vi "Measure Delta Mode.vi"(0 "Current Source Reference In":string="6221_GPIB12", 1 "Current Level (A)":dbl=1e-05, 2 "Current Range (A)":dbl=0.0001 format="%.2e", 3 "Current Source Compliance (V)":dbl=10.0 min=-1050.0 max=1050.0 step=1.0 format="%.4f", 5 "Voltmeter Reference In":refnum<visa-resource-name>="GPIB0::7::INSTR", 9 "Error in Current Source":errorcluster, 11 "Error In Voltmeter":errorcluster, 13 "Voltmeter Wait (ms)":u32=400) -> (4 "Current Source Reference Out":refnum<k15>, 6 "Voltmeter Reference Out":refnum<visa-resource-name>="GPIB0::7::INSTR", 8 "Resistance":dbl=1.1800557999999999, 10 "Error Out Current Source":errorcluster, 15 "Error Out Voltmeter":errorcluster)   [LabVIEW 2020]
uses:
  <instrlib>/Keithley 2182/Keithley 2182.lvlib
panel:
  out "Pulse Down Voltage":dbl=-2.087828e-05
  out "Pulse Up Voltage":dbl=2.722836e-06
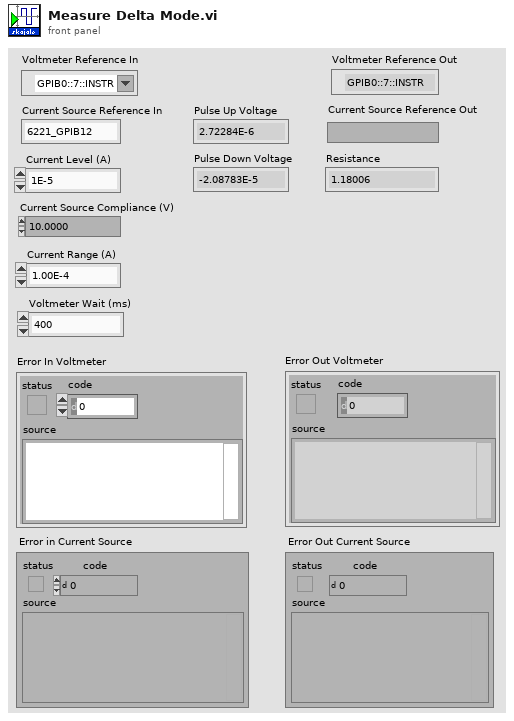
[diagram p1: front panel]
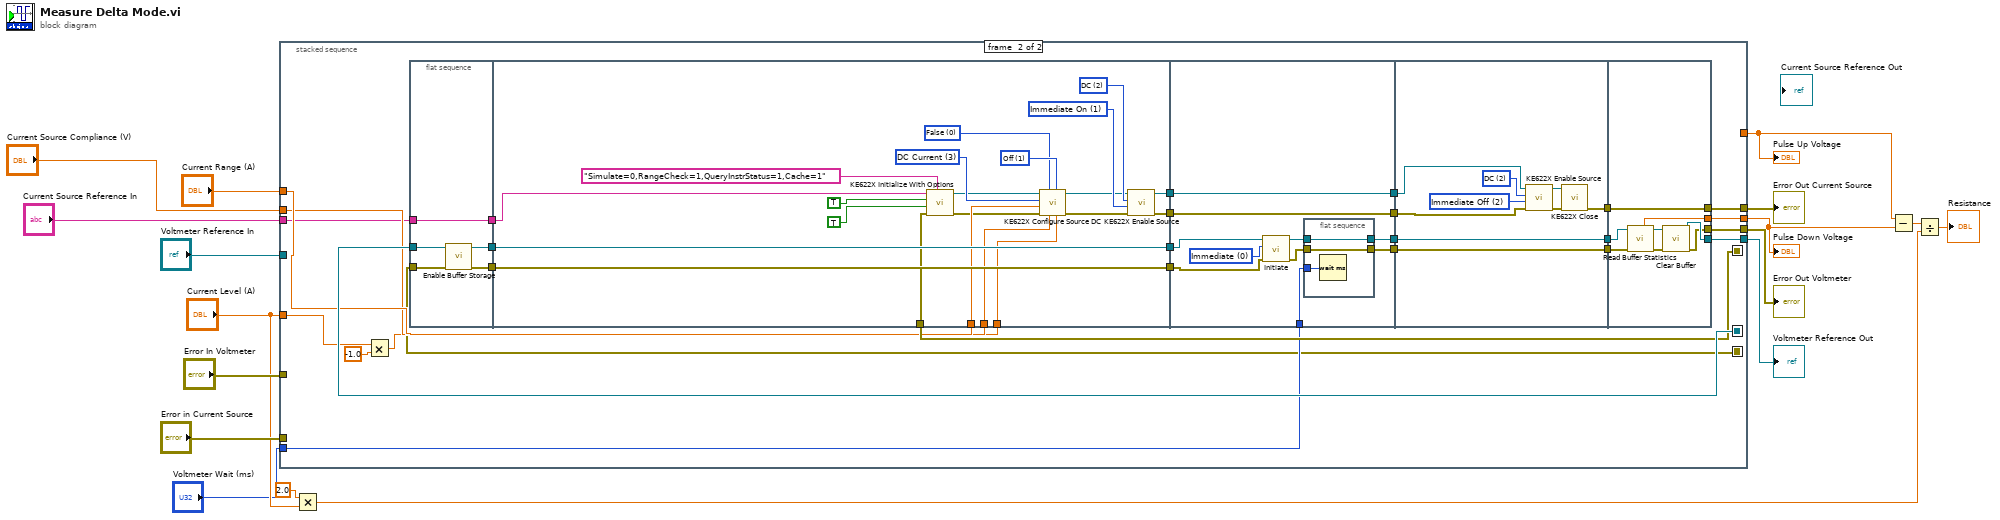
[diagram p0: block diagram]
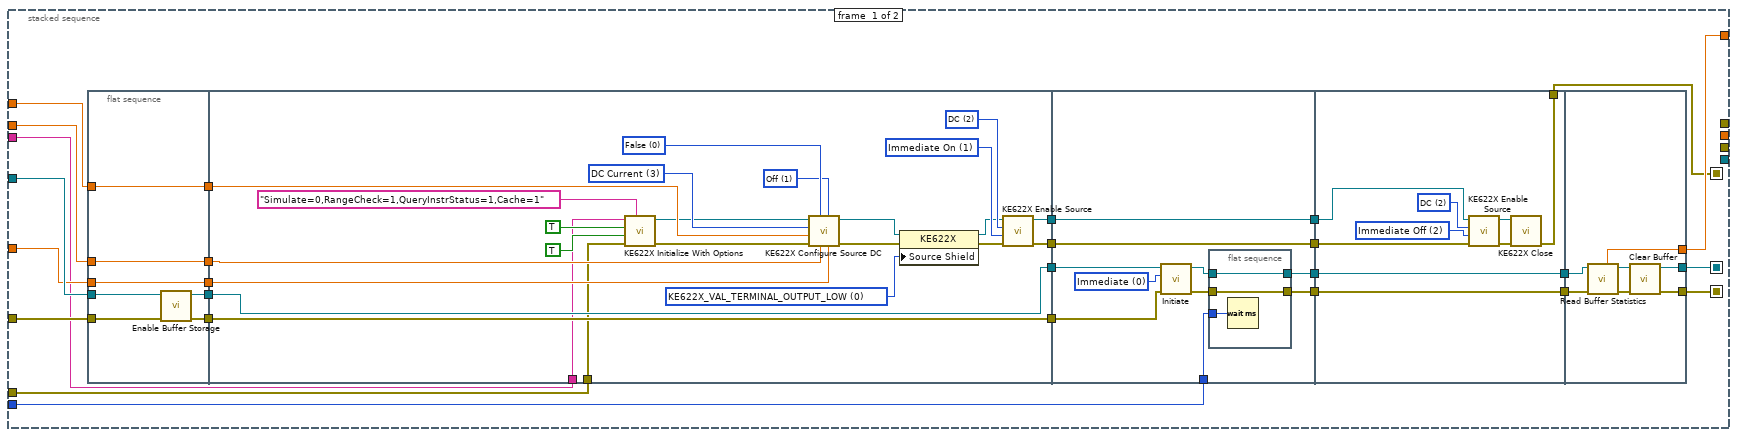
[diagram p2: hidden frame]
diagram:
  n1 = stacked-sequence {
    seq-local: [w31 _] -> [_ w120]
    seq-local: [w30 _] -> [_ w106]
    seq-local: [w29 _] -> [_ w119]
    tunnel: [w32 _] -> w15
    tunnel: [_ w118] -> w14
    tunnel: [_ w117] -> w4
    tunnel: [_ w116] -> w17
    tunnel: [_ w114] -> w16
    tunnel: "Voltmeter Reference In" -> [w28 _]
    tunnel: "Current Range (A)" -> [w26 w113]
    tunnel: "Error in Current Source" -> [w25 _]
    tunnel: "Current Source Compliance (V)" -> [w23 w112]
    tunnel: "Current Level (A)" -> [w22 w111]
    tunnel: "Error In Voltmeter" -> [w20 _]
    tunnel: "Voltmeter Wait (ms)" -> [w19 w108]
    tunnel: "Current Source Reference In" -> [w18 w105]
    frame #0 {
      n2 = flat-sequence {
        tunnel: [w51] -> w44
        tunnel: [w50] -> w43
        tunnel: w28 -> [w49]
        tunnel: w26 -> [w48]
        tunnel: [w48] -> w27
        tunnel: w23 -> [w47]
        tunnel: [w47] -> w24
        tunnel: w22 -> [w46]
        tunnel: [w46] -> w21
        tunnel: w20 -> [w45]
        tunnel: [w75] -> w42
        tunnel: w44 -> [w75]
        tunnel: [w74] -> w41
        tunnel: w43 -> [w74]
        tunnel: [w71] -> w40
        tunnel: [w70] -> w39
        tunnel: w27 -> [w66]
        tunnel: w25 -> [w56]
        tunnel: w24 -> [w65]
        tunnel: w21 -> [w64]
        tunnel: w18 -> [w52]
        tunnel: w42 -> [w83]
        tunnel: w41 -> [w82]
        tunnel: [w80] -> w38
        tunnel: [w79] -> w37
        tunnel: [w78] -> w36
        tunnel: w40 -> [w78]
        tunnel: [w77] -> w35
        tunnel: w39 -> [w77]
        tunnel: w19 -> [w76]
        tunnel: [w97] -> w34
        tunnel: w38 -> [w97]
        tunnel: [w96] -> w33
        tunnel: w37 -> [w96]
        tunnel: w36 -> [w95]
        tunnel: w35 -> [w94]
        tunnel: [w89] -> w29
        tunnel: w34 -> [w104]
        tunnel: w33 -> [w102]
        tunnel: [w100] -> w31
        tunnel: [w98] -> w32
        tunnel: [w99] -> w30
        frame #0 {
          n3 = call <instrlib>:"Enable Buffer Storage.vi"("error in (no error)"=w45, "VISA resource name"=w49) -> ("error out"=w50:errorcluster, "VISA resource name out"=w51:refnum<visa-resource-name>)  [unwired: 8 in]
        }
        frame #1 {
          w59 = 0 items=["KE622X_VAL_TERMINAL_OUTPUT_LOW", "KE622X_VAL_TERMINAL_GUARD"] ("System Settings:Source Shield")
          w67 = 3 items=["DC Current"=3] ("function")
          w68 = 1 items=["Off"=1, "HighZ"=3] ("standby mode")
          w69 = u16 0 items=["False"] ("enable pulsing")
          w72 = 1 items=["Immediate On"=1, "Immediate Off"=2, "Immediate Standby"=4, "Auto Sync Enabled"=65536, "Auto Sync Disabled"=131072, "Abort On Compliance Enabled"=16777216, "Abort On Compliance Disabled"=33554432] ("output action")
          w73 = 2 items=["Bias"=1, "Custom"=8, "DC"=2, "Sweep"=4, "Pulse Gen"=16, "Standard Waveform"=32, "Arbitrary Waveform"=64] ("generator")
          n4 = call <instrlib>:"KE622X Initialize With Options.vi"("option string"="Simulate=0,RangeCheck=1,QueryInstrStatus=1,Cache=1", "error in (no error)"=w56, "reset device"=TRUE, "id query"=TRUE, "resource name"=w52) -> ("error out"=w55:errorcluster, "instrument handle out"=w54:refnum<k15>)  [unwired: 5 in]
          n5 = call <instrlib>:"KE622X Configure Source DC.vi"("level"=w64, "standby mode"=w68, "compliance limit"=w65, "enable pulsing"=w69, "error in (no error)"=w55, "range"=w66, "function"=w67, "instrument handle"=w54) -> ("error out"=w62:errorcluster, "instrument handle out"=w63:refnum<k15>)  [unwired: 2 in]
          n6 = property class="KE622X"(reference=w63, error in=w62, "Source Shield"=w59) -> (reference out=w61:refnum<k15>, error out=w60:errorcluster)
          n7 = call <instrlib>:"KE622X Enable Source.vi"("error in (no error)"=w60, "output action"=w72, "generator"=w73, "instrument handle"=w61) -> ("error out"=w70:errorcluster, "instrument handle out"=w71:refnum<k15>)  [unwired: 6 in]
        }
        frame #2 {
          w81 = 0 items=["Immediate", "Continuous"] ("Initiate Type (0: Immediate)")
          n8 = call <instrlib>:"Initiate.vi"("error in (no error)"=w82, "Initiate Type (0: Immediate)"=w81, "VISA resource name"=w83) -> ("error out"=w85:errorcluster, "VISA resource name out"=w84:refnum<visa-resource-name>)  [unwired: 7 in]
          n9 = flat-sequence {
            tunnel: w76 -> [w88]
            tunnel: [w87] -> w79
            tunnel: w85 -> [w87]
            tunnel: [w86] -> w80
            tunnel: w84 -> [w86]
            frame #0 {
              n10 = Wait (ms)(milliseconds to wait=w88) -> ()  [unwired: 1 out]
            }
          }
        }
        frame #3 {
          w92 = 2 items=["Immediate On"=1, "Immediate Off"=2, "Immediate Standby"=4, "Auto Sync Enabled"=65536, "Auto Sync Disabled"=131072, "Abort On Compliance Enabled"=16777216, "Abort On Compliance Disabled"=33554432] ("output action")
          w93 = 2 items=["Bias"=1, "Custom"=8, "DC"=2, "Sweep"=4, "Pulse Gen"=16, "Standard Waveform"=32, "Arbitrary Waveform"=64] ("generator")
          n11 = call <instrlib>:"KE622X Enable Source.vi"("error in (no error)"=w94, "output action"=w92, "generator"=w93, "instrument handle"=w95) -> ("error out"=w90:errorcluster, "instrument handle out"=w91:refnum<k15>)  [unwired: 6 in]
          n12 = call <userlib>:"KE622X Close.vi"("error in (no error)"=w90, "instrument handle"=w91) -> ("error out"=w89:errorcluster)  [unwired: 9 in]
        }
        frame #4 {
          n13 = call <instrlib>:"Read Buffer Statistics.vi"("error in (no error)"=w102, "VISA resource name"=w104) -> ("error out"=w101:errorcluster, "VISA resource name out"=w103:refnum<visa-resource-name>, "Mean"=w98:dbl)  [unwired: 4 in, 3 out]
          n14 = call <instrlib>:"Clear Buffer.vi"("error in (no error)"=w101, "VISA resource name"=w103) -> ("error out"=w99:errorcluster, "VISA resource name out"=w100:refnum<visa-resource-name>)  [unwired: 8 in]
        }
      }
    }
    frame #1 {
      n15 = Multiply(x=w111, y=-1.0) -> (x*y=w109:dbl)
      n16 = flat-sequence {
        tunnel: [w137] -> w132
        tunnel: [w136] -> w131
        tunnel: w120 -> [w135]
        tunnel: w106 -> [w134]
        tunnel: [w133] -> w107
        tunnel: w105 -> [w133]
        tunnel: [w158] -> w130
        tunnel: w132 -> [w158]
        tunnel: [w157] -> w129
        tunnel: w131 -> [w157]
        tunnel: [w154] -> w128
        tunnel: [w153] -> w127
        tunnel: w119 -> [w142]
        tunnel: w113 -> [w147]
        tunnel: w112 -> [w146]
        tunnel: w109 -> [w145]
        tunnel: w107 -> [w143]
        tunnel: w130 -> [w166]
        tunnel: w129 -> [w165]
        tunnel: [w163] -> w126
        tunnel: [w162] -> w125
        tunnel: [w161] -> w124
        tunnel: w128 -> [w161]
        tunnel: [w160] -> w123
        tunnel: w127 -> [w160]
        tunnel: w108 -> [w159]
        tunnel: [w180] -> w122
        tunnel: w126 -> [w180]
        tunnel: [w179] -> w121
        tunnel: w125 -> [w179]
        tunnel: w124 -> [w178]
        tunnel: w123 -> [w177]
        tunnel: [w172] -> w115
        tunnel: w122 -> [w188]
        tunnel: w121 -> [w186]
        tunnel: [w184] -> w117
        tunnel: [w183] -> w116
        tunnel: [w181] -> w118
        tunnel: [w182] -> w114
        tunnel: w115 -> [w182]
        frame #0 {
          n17 = call <instrlib>:"Enable Buffer Storage.vi"("error in (no error)"=w134, "VISA resource name"=w135) -> ("error out"=w136:errorcluster, "VISA resource name out"=w137:refnum<visa-resource-name>)  [unwired: 8 in]
        }
        frame #1 {
          w148 = 3 items=["DC Current"=3] ("function")
          w151 = u16 0 items=["False"] ("enable pulsing")
          w152 = 1 items=["Off"=1, "HighZ"=3] ("standby mode")
          w155 = 1 items=["Immediate On"=1, "Immediate Off"=2, "Immediate Standby"=4, "Auto Sync Enabled"=65536, "Auto Sync Disabled"=131072, "Abort On Compliance Enabled"=16777216, "Abort On Compliance Disabled"=33554432] ("output action")
          w156 = 2 items=["Bias"=1, "Custom"=8, "DC"=2, "Sweep"=4, "Pulse Gen"=16, "Standard Waveform"=32, "Arbitrary Waveform"=64] ("generator")
          n18 = call <instrlib>:"KE622X Initialize With Options.vi"("option string"="Simulate=0,RangeCheck=1,QueryInstrStatus=1,Cache=1", "error in (no error)"=w142, "reset device"=TRUE, "id query"=TRUE, "resource name"=w143) -> ("error out"=w138:errorcluster, "instrument handle out"=w139:refnum<k15>)  [unwired: 5 in]
          n19 = call <instrlib>:"KE622X Configure Source DC.vi"("level"=w145, "standby mode"=w152, "compliance limit"=w146, "enable pulsing"=w151, "error in (no error)"=w138, "range"=w147, "function"=w148, "instrument handle"=w139) -> ("error out"=w149:errorcluster, "instrument handle out"=w150:refnum<k15>)  [unwired: 2 in]
          n20 = call <instrlib>:"KE622X Enable Source.vi"("error in (no error)"=w149, "output action"=w155, "generator"=w156, "instrument handle"=w150) -> ("error out"=w153:errorcluster, "instrument handle out"=w154:refnum<k15>)  [unwired: 6 in]
        }
        frame #2 {
          w164 = 0 items=["Immediate", "Continuous"] ("Initiate Type (0: Immediate)")
          n21 = call <instrlib>:"Initiate.vi"("error in (no error)"=w165, "Initiate Type (0: Immediate)"=w164, "VISA resource name"=w166) -> ("error out"=w168:errorcluster, "VISA resource name out"=w167:refnum<visa-resource-name>)  [unwired: 7 in]
          n22 = flat-sequence {
            tunnel: w159 -> [w171]
            tunnel: [w170] -> w162
            tunnel: w168 -> [w170]
            tunnel: [w169] -> w163
            tunnel: w167 -> [w169]
            frame #0 {
              n23 = Wait (ms)(milliseconds to wait=w171) -> ()  [unwired: 1 out]
            }
          }
        }
        frame #3 {
          w175 = 2 items=["Immediate On"=1, "Immediate Off"=2, "Immediate Standby"=4, "Auto Sync Enabled"=65536, "Auto Sync Disabled"=131072, "Abort On Compliance Enabled"=16777216, "Abort On Compliance Disabled"=33554432] ("output action")
          w176 = 2 items=["Bias"=1, "Custom"=8, "DC"=2, "Sweep"=4, "Pulse Gen"=16, "Standard Waveform"=32, "Arbitrary Waveform"=64] ("generator")
          n24 = call <instrlib>:"KE622X Enable Source.vi"("error in (no error)"=w177, "output action"=w175, "generator"=w176, "instrument handle"=w178) -> ("error out"=w173:errorcluster, "instrument handle out"=w174:refnum<k15>)  [unwired: 6 in]
          n25 = call <userlib>:"KE622X Close.vi"("error in (no error)"=w173, "instrument handle"=w174) -> ("error out"=w172:errorcluster)  [unwired: 9 in]
        }
        frame #4 {
          n26 = call <instrlib>:"Read Buffer Statistics.vi"("error in (no error)"=w186, "VISA resource name"=w188) -> ("error out"=w185:errorcluster, "VISA resource name out"=w187:refnum<visa-resource-name>, "Mean"=w181:dbl)  [unwired: 4 in, 3 out]
          n27 = call <instrlib>:"Clear Buffer.vi"("error in (no error)"=w185, "VISA resource name"=w187) -> ("error out"=w183:errorcluster, "VISA resource name out"=w184:refnum<visa-resource-name>)  [unwired: 8 in]
        }
      }
    }
  }
  "Voltmeter Reference Out" <- w4
  "Error Out Voltmeter" <- w17
  "Pulse Up Voltage" <- w15
  "Error Out Current Source" <- w16
  "Pulse Down Voltage" <- w14
  n28 = Multiply(x=2.0, y="Current Level (A)") -> (x*y=w3:dbl)
  n29 = Subtract(x=w15, y=w14) -> (x-y=w13:dbl)
  n30 = Divide(x=w13, y=w3) -> (x/y=→"Resistance":dbl)
